vi "AO-loop.vi"(8 "错误输入（无错误）":errorcluster, 11 "Status":T1 {"Setting"."X Pos." scale=-2.0..2.0; "Setting"."Y Pos." scale=-2.0..2.0}) -> (0 "Error out":errorcluster={"status"=TRUE, "code"=-200099, "source"="DAQmx Create Channel (AI-Voltage-Basic).vi:1780001<append>\n<B>任务名称: </B>_unnamedTask<1>"} caption="错误输入（无错误）")   [LabVIEW 2013]
uses:
  init & communication/init-status.ctl
  init & communication/Setting.ctl
  init & communication/event-package.ctl
  init & communication/Event1.ctl
  init & communication/data-package.ctl
  init & communication/Event.ctl
  <vilib>/Utility/error.llb/DialogType.ctl
  <vilib>/DAQmx/write.llb/DAQmx Write (Analog 1D Wfm NChan NSamp).vi
  <vilib>/DAQmx/create/channels.llb/DAQmx Create Channel (AO-Voltage-Basic).vi
  <vilib>/DAQmx/configure/timing.llb/DAQmx Timing (Sample Clock).vi
  <vilib>/DAQmx/configure/trigger.llb/DAQmx Start Trigger (Digital Edge).vi
  <vilib>/DAQmx/miscellaneous.llb/DAQmx Fill In Error Info.vi
  <resource>/objmgr/daqmx.rc
panel:
  out "波形图":waveform(dbl)[](graph)
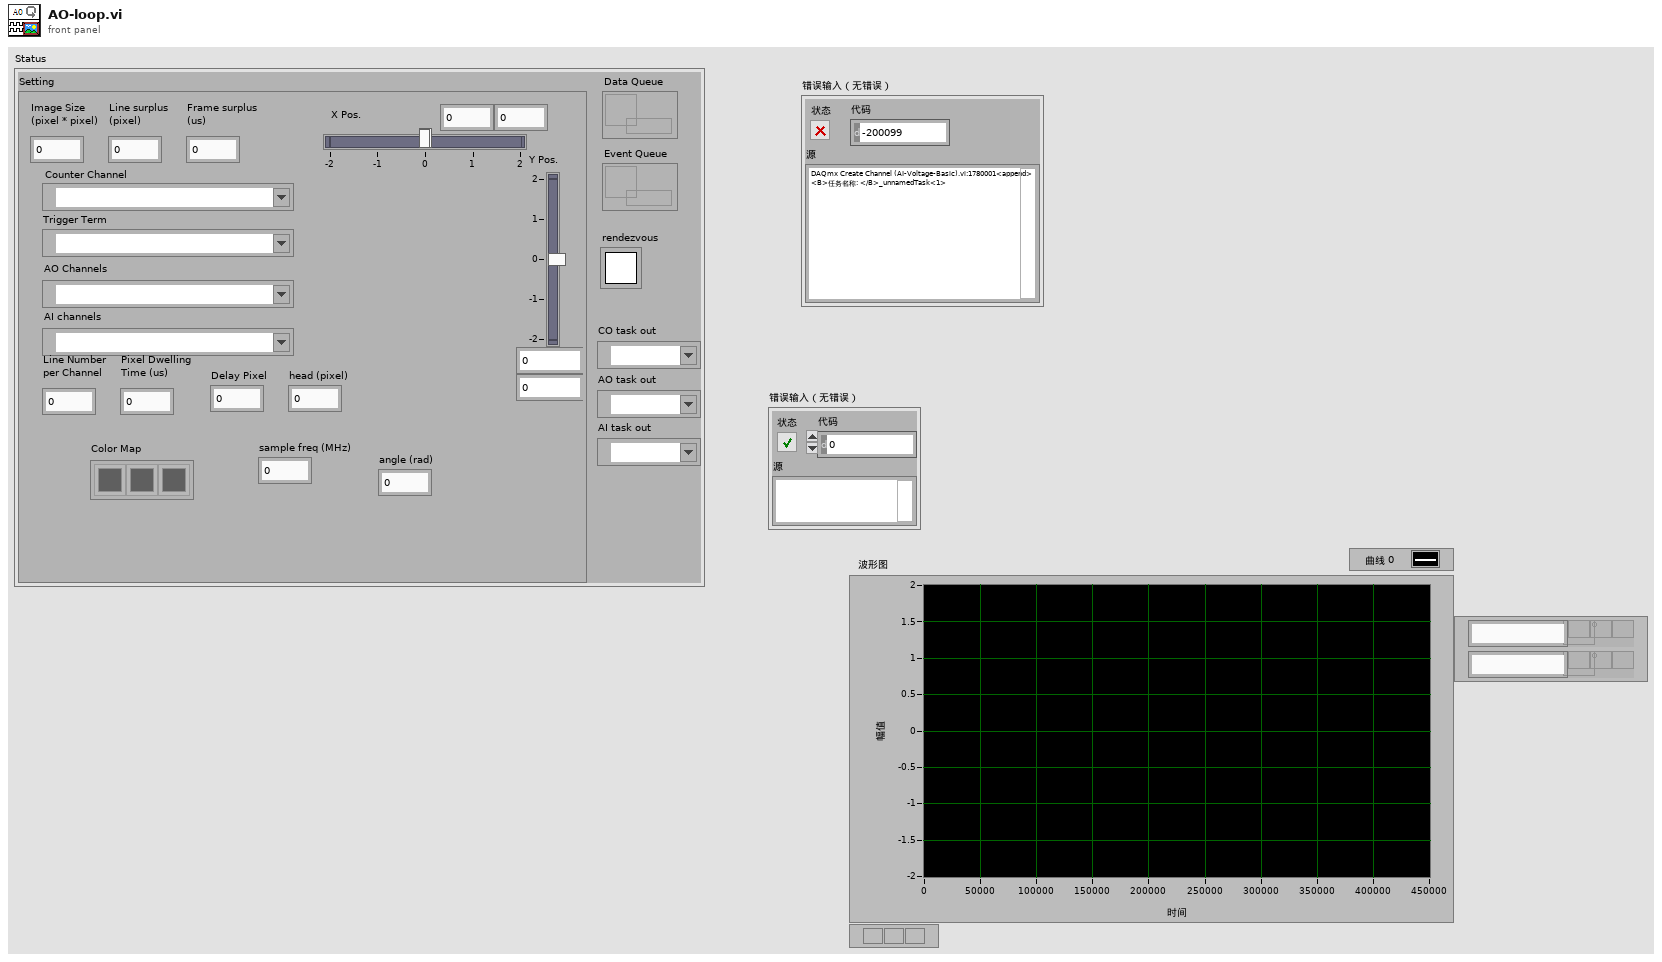
[diagram p1: front panel]
types:
  T1 = typedef "init-status.ctl" = cluster{"Setting":T2, "Event Queue":refnum<queue>, "Data Queue":refnum<queue>, "rendezvous":T3, "CO task out":refnum<k21>, "AO task out":refnum<k21>, "AI task out":refnum<k21>}
  T2 = typedef "Setting.ctl" = cluster{"Image Size\n(pixel * pixel)":i32, "Counter Channel":tag, "Trigger Term":tag, "AO Channels":tag, "Y Pos.":cluster{dbl, dbl}, "X Pos.":cluster{dbl, dbl}, "Line surplus\n(pixel)":i32, "Frame surplus\n(us)":i32, "AI channels":tag, "Line Number\nper Channel":i32, "Delay Pixel":i32, "Pixel Dwelling\nTime (us)":i32, "Color Map":u32[], "head (pixel)":i32, "sample freq (MHz)":dbl, "angle (rad)":dbl}
  T3 = typedef "Rendezvous RefNum" = refnum<k1>
  T4 = typedef "DialogType.ctl" = u16
  T5 = typedef "Event1.ctl" = enum16{"null", "stop AI", "stop AO", "stop Imaging", "stop Counter", "save sheet", "restart", "save tiff", "gain/offset changed", "save multiple tiffs"}
  T6 = typedef "event-package.ctl" = cluster{"Event":T5, "Data":string}
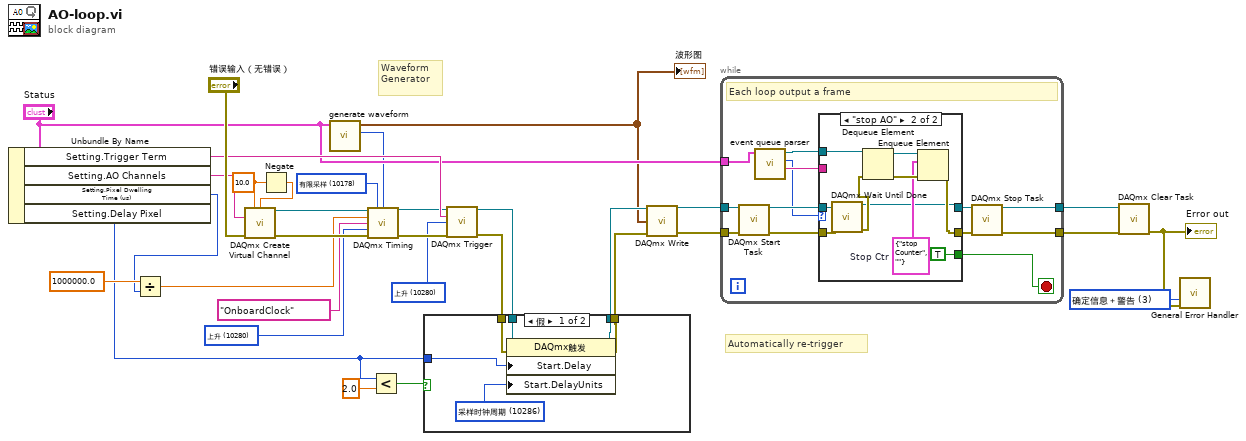
[diagram p0: block diagram]
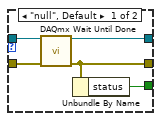
[diagram p3: hidden frame]
diagram:
  w13 = T4 3 items=["无对话框", "确定信息", "继续或停止信息", "确定信息＋警告", "继续/停止+警告"] ("type of dialog (OK msg:1)")
  w19 = 10280 items=["上升"=10280, "下降"=10171] ("edge")
  w22 = 10178 items=["有限采样"=10178, "连续采样"=10123, "硬件定时单点"=12522] ("sample mode")
  w23 = 10280 items=["上升"=10280, "下降"=10171] ("active edge")
  w25 = 10.0
  # "Waveform\nGenerator"
  # "Automatically re-trigger"
  n1 = Unbundle By Name("Status") -> ("Setting.Trigger Term"=w30:tag, "Setting.AO Channels"=w21:tag, "Setting.Pixel Dwelling\nTime (us)"=w6:i32, "Setting.Delay Pixel"=w2:i32)
  n2 = Divide(x=1000000.0 ("rate"), y=w6) -> (x/y=w5:dbl)
  n3 = Negate(x=w25) -> (-x=w26:dbl)
  n4 = call-poly <vilib>:"DAQmx Create Virtual Channel.vi"("maximum value"=w25, "minimum value"=w26, "physical channels"=w21, "error in"="错误输入（无错误）") -> ("task out"=w31:refnum<k21>, "error out"=w27:errorcluster)  [unwired: 10 in]
  n5 = call "generate waveform.vi"("Status"="Status") -> ("sample number"=w12:i32, "波形图"=w1:waveform(dbl)[])  [unwired: 9 in]
  "波形图" <- w1
  n6 = call-poly <vilib>:"DAQmx Timing.vi"("task/channels in"=w31, "sample mode"=w22, "samples per channel"=w12, "rate"=w5, "source"=tag "OnboardClock", "active edge"=w23, "error in"=w27) -> ("task out"=w29:refnum<k21>, "error out"=w28:errorcluster)  [unwired: 7 in]
  n7 = Less?(x=w2, y=2.0) -> (x < y?=w3:bool)
  n8 = call-poly <vilib>:"DAQmx Trigger.vi"("task/channels in"=w29, "source"=w30, "edge"=w19, "error in"=w28) -> ("task out"=w11:refnum<k21>, "error out"=w9:errorcluster)  [unwired: 10 in]
  n9 = case shown="假" w3 {
    tunnel: w11 -> [w38 w40]
    tunnel: [w37 w40] -> w10
    tunnel: w9 -> [w36 w39]
    tunnel: [w35 w39] -> w8
    tunnel: w2 -> [w34 _]
    frame False {
      w33 = 10286 items=["采样时钟周期"=10286, "秒"=10364, "时钟滴答"=10304] ("Start.DelayUnits")
      n10 = property class="DAQmx触发"(reference=w38, error in=w36, "Start.Delay"=w34, "Start.DelayUnits"=w33) -> (reference out=w37:refnum<k21>, error out=w35:errorcluster)
    }
    frame True {
    }
  }
  n11 = call-poly <vilib>:"DAQmx Write.vi"("task/channels in"=w10, "data"=w1, "error in"=w8) -> ("task out"=w18:refnum<k21>, "error out"=w17:errorcluster)  [unwired: 10 in, 1 out]
  n12 = while {
    tunnel: "Status" -> [w44]
    tunnel: w18 -> [w52]
    tunnel: w17 -> [w51]
    tunnel: [w50] -> w15
    tunnel: [w49] -> w14
    stop <- w53 stop-if-true
    # "Each loop output a frame"
    n13 = call <vilib>:"DAQmx Start Task.vi"("task/channels in"=w52, "error in"=w51) -> ("task out"=w48:refnum<k21>, "error out"=w45:errorcluster)  [unwired: 12 in]
    n14 = call "event queue parser.vi"("Status"=w44) -> ("Data"=w42:string, "Event"=w41:T5, "队列输出"=w43:refnum<queue>)  [unwired: 8 in]
    n15 = case shown="\"stop AO\"" w41 {
      tunnel: [w54 TRUE] -> w53
      tunnel: w48 -> [w58 w62]
      tunnel: [w57 w59] -> w47
      tunnel: [w55 w63] -> w46
      tunnel: w45 -> [w56 w61]
      tunnel: w43 -> [_ w68]
      tunnel: w42 -> [_ _]
      frame "null", Default {
        n16 = call <vilib>:"DAQmx Wait Until Done.vi"("task/channels in"=w58, "error in"=w56) -> ("task out"=w57:refnum<k21>, "error out"=w55:errorcluster)  [unwired: 12 in]
        n17 = Unbundle By Name(w55) -> ("status"=w54:bool)
      }
      frame "stop AO" {
        w65 = T6 {"Event"=enum."stop Counter", "Data"=""}  # Stop Ctr
        n18 = call <vilib>:"DAQmx Wait Until Done.vi"("task/channels in"=w62, "error in"=w61) -> ("task out"=w59:refnum<k21>, "error out"=w60:errorcluster)  [unwired: 12 in]
        n19 = Dequeue Element(queue=w68, error in (no error)=w60) -> (queue out=w67:refnum<queue>, error out=w66:errorcluster)  [unwired: 1 in, 2 out]
        n20 = Enqueue Element(queue=w67, element=w65, error in (no error)=w66) -> (error out=w63:errorcluster)  [unwired: 1 in, 2 out]
      }
    }
    n21 = call <vilib>:"DAQmx Stop Task.vi"("task/channels in"=w47, "error in"=w46) -> ("task out"=w50:refnum<k21>, "error out"=w49:errorcluster)  [unwired: 12 in]
  }
  n22 = call <vilib>:"DAQmx Clear Task.vi"("task in"=w15, "error in"=w14) -> ("error out"=w16:errorcluster)  [unwired: 13 in]
  "Error out" <- w16
  n23 = call <vilib>:"General Error Handler.vi"("type of dialog (OK msg:1)"=w13, "error in (no error)"=w16) -> ()  [unwired: 9 in, 5 out]
